vi "uTransport_BlockingTwoWayMsg.vi"(6 "timeout in ms (5000)":i32=5000, 8 "error in (no error)":errorcluster, 9 "Data":refnum<class "uData.lvclass">, 10 "Command":string, 11 "uTransport in":refnum<class "uTransport.lvclass">) -> (0 "error out":errorcluster, 1 "Reply":refnum<class "uData.lvclass">)   [LabVIEW 2021, in "uFramework.lvlib" / "uTransport.lvclass"]
doc: "Use to Send a message and wait for a synchronous reply.\nReturns error 550011 on timeout."
uses:
  uTransport.lvclass
  Bin/uData.lvlibp/uData.lvclass
  uTransport_Queue/uTransport_Queue.lvclass/uTransport_Queue.ctl
  uMsg/uMsg.lvclass/uMsg.ctl
  uMsg/uMsg Update Timestamp.vi
  uTransport_Queue/uTransport_Queue.lvclass
  U:/Projects/uFramework/Src/uFramework/uTransport/uTransport.lvclass
  <vilib>/Utility/error.llb/Error Cluster From Error Code.vi
  uMsg/uMsg.lvclass
  <vilib>/ErrorRing/Error Ring.xnode
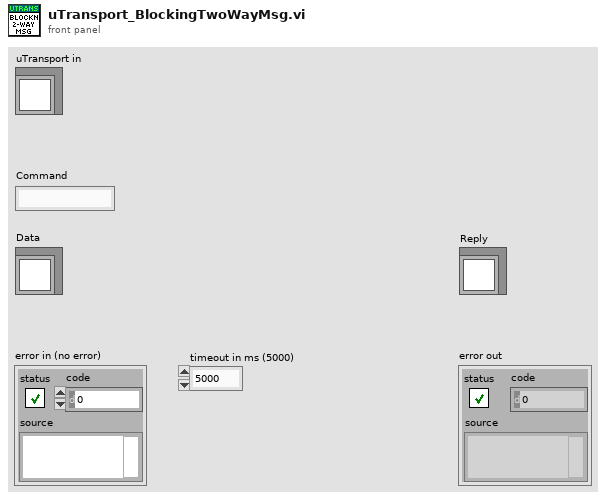
[diagram p1: front panel]
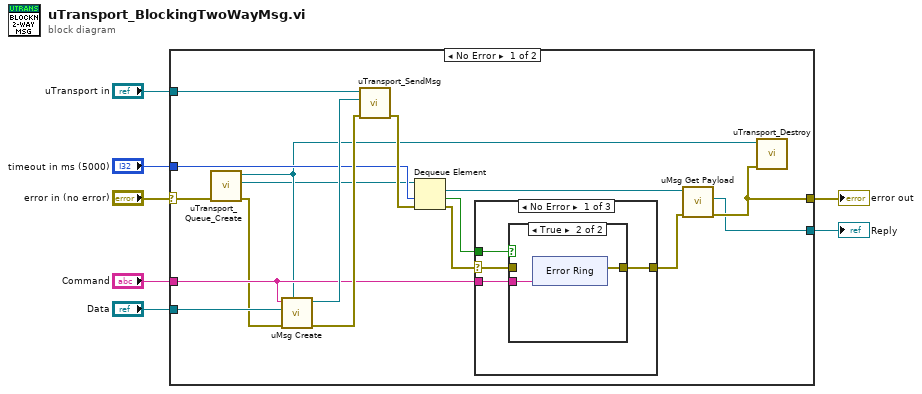
[diagram p0: block diagram]
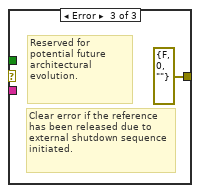
[diagram p4: hidden frame]
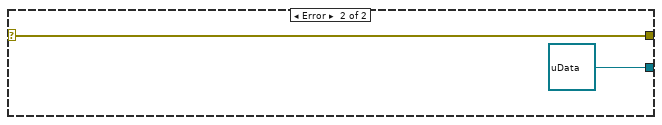
[diagram p5: hidden frame]
diagram:
  n1 = case shown="No Error" "error in (no error)" {
    selector: "error in (no error)" -> [w20 w42]
    tunnel: "Command" -> [w17 _]
    tunnel: "uTransport in" -> [w22 _]
    tunnel: "Data" -> [w19 _]
    tunnel: "timeout in ms (5000)" -> [w15 _]
    tunnel: [w12 w42] -> w3
    tunnel: [w11 refnum<class "uData.lvclass"> refnum ("Msg")] -> w1
    frame No Error {
      n2 = call "uTransport_Queue_Create.vi"("error in (no error)"=w20) -> ("error out"=w16:errorcluster, "queue"=w10:refnum<queue>, "uTransport_Queue out"=w14:refnum<class "uTransport_Queue.lvclass">)  [unwired: 8 in]
      n3 = call "uMsg Create.vi"("Reply Transport"=w14, "error in (no error)"=w16, "Payload"=w19, "CMD"=w17) -> ("error out"=w23:errorcluster, "uMsg out"=w18:refnum<class "uMsg.lvclass">)  [unwired: 6 in]
      n4 = call "uTransport_SendMsg.vi"("error in (no error)"=w23, "Msg"=w18, "uTransport in"=w22) -> ("error out"=w24:errorcluster)  [unwired: 7 in, 1 out]
      n5 = Dequeue Element(queue=w10, timeout in ms (-1)=w15, error in (no error)=w24) -> (element=w9:refnum<class "uMsg.lvclass">, timed out?=w8:bool, error out=w21:errorcluster)  [unwired: 1 out]
      n6 = case shown="No Error" w21 {
        selector: w21 -> [w25 w39 _]
        tunnel: [w27 w39 errorcluster {"status"=FALSE, "code"=0, "source"=""} ("error IO")] -> w13
        tunnel: w17 -> [w28 _ _]
        tunnel: w8 -> [w26 _ _]
        frame No Error {
          n7 = case shown="True" w26 {
            tunnel: w28 -> [_ w31]
            tunnel: [w29 w30] -> w27
            tunnel: w25 -> [w29 _]
            frame False {
            }
            frame True {
              n8 = xnode "Error Ring"("parameter 0"=w31) -> ("error out"=w30:errorcluster)
            }
          }
        }
        frame Default {
        }
        frame Error {
          # "Reserved for potential future architectural evolution."
          # "Clear error if the reference has been released due to external shutdown sequence initiated."
        }
      }
      n9 = call "uMsg Get Payload.vi"("error in (no error)"=w13, "uMsg in"=w9) -> ("error out"=w12:errorcluster, "uData"=w11:refnum<class "uData.lvclass">)  [unwired: 7 in, 1 out]
      n10 = call-dynamic "uTransport_Destroy.vi"("error in (no error)"=w12, "uTransport_Queue in"=w14) -> ()  [unwired: 9 in, 1 out]
    }
    frame Error {
    }
  }
  "error out" <- w3
  "Reply" <- w1
